vi "SwerveDriveFace.vi"(0 "Strafe Joystick Axes":cluster{"X":dbl, "Y":dbl}, 1 "Face Joystick Axes":cluster{"X":dbl, "Y":dbl}, 3 "Face PID Gains":T9 {"derivative time (Td, min)" format="%.3f"; "integral time (Ti, min)" format="%.3f"; "proportional gain (Kc)" format="%.3f"}, 4 "Angle (degrees; 0 = right)":dbl, 5 "error in (no error)":errorcluster, 6 "Strafe Multiplier":dbl, 7 "Steering Motor Refs":T1[](array[typedef]), 8 "Rotation Multiplier":dbl, 9 "Speed Motor Refs":T1[](array[typedef]), 10 "Max Wheel Speed":dbl) -> (14 "Steering Motor Setpoints":dbl[](array[numeric]), 15 "Speed Motor Setpoints":dbl[](array[numeric]), 16 "Speed Chart":cluster{dbl, "Encoder Velocity":dbl}[](graph), 19 "error out":errorcluster)   [LabVIEW 2015, in "Team900SwerveDrive.lvlib"]
uses:
  Team900SwerveDrive.lvlib
  <vilib>/Rock Robotics/WPI/MotorControl/WPI_MotorControlDeviceRef.ctl
  <vilib>/Rock Robotics/WPI/MotorControl/WPI_MotorControlType.ctl
  <vilib>/Rock Robotics/SystemInterfaces/DIO/FPGA_DIOPWMChannel.ctl
  <vilib>/Rock Robotics/WPI/PWM/WPI_PWMDeadband.ctl
  <vilib>/Rock Robotics/WPI/CAN/Jaguar/SubVIs/WPI_CANJaguar_ControlMode.ctl
  <vilib>/Rock Robotics/WPI/CAN/TalonSRX/WPI_CANTalonSRX_APIControlMode.ctl
  <vilib>/addons/control/pid/pid.llb/PID Control Input Filter (DBL).vi
  <vilib>/addons/control/pid/pid.llb/PID (DBL).vi
  <vilib>/addons/control/pid/NI_PID_pid.lvlib
panel:
  out "diff.":dbl
  out "Waveform Chart":T8(graph)
  out "Robot Heading":dbl(knob) scale=3.1416..-3.1416
  out "Joystick Angle":dbl(knob) scale=3.1416..-3.1416
  # "A version of SwerveDrive.vi which only takes\ntwo joysticks, one for strafe and one to use \nas a setpoint for angle"
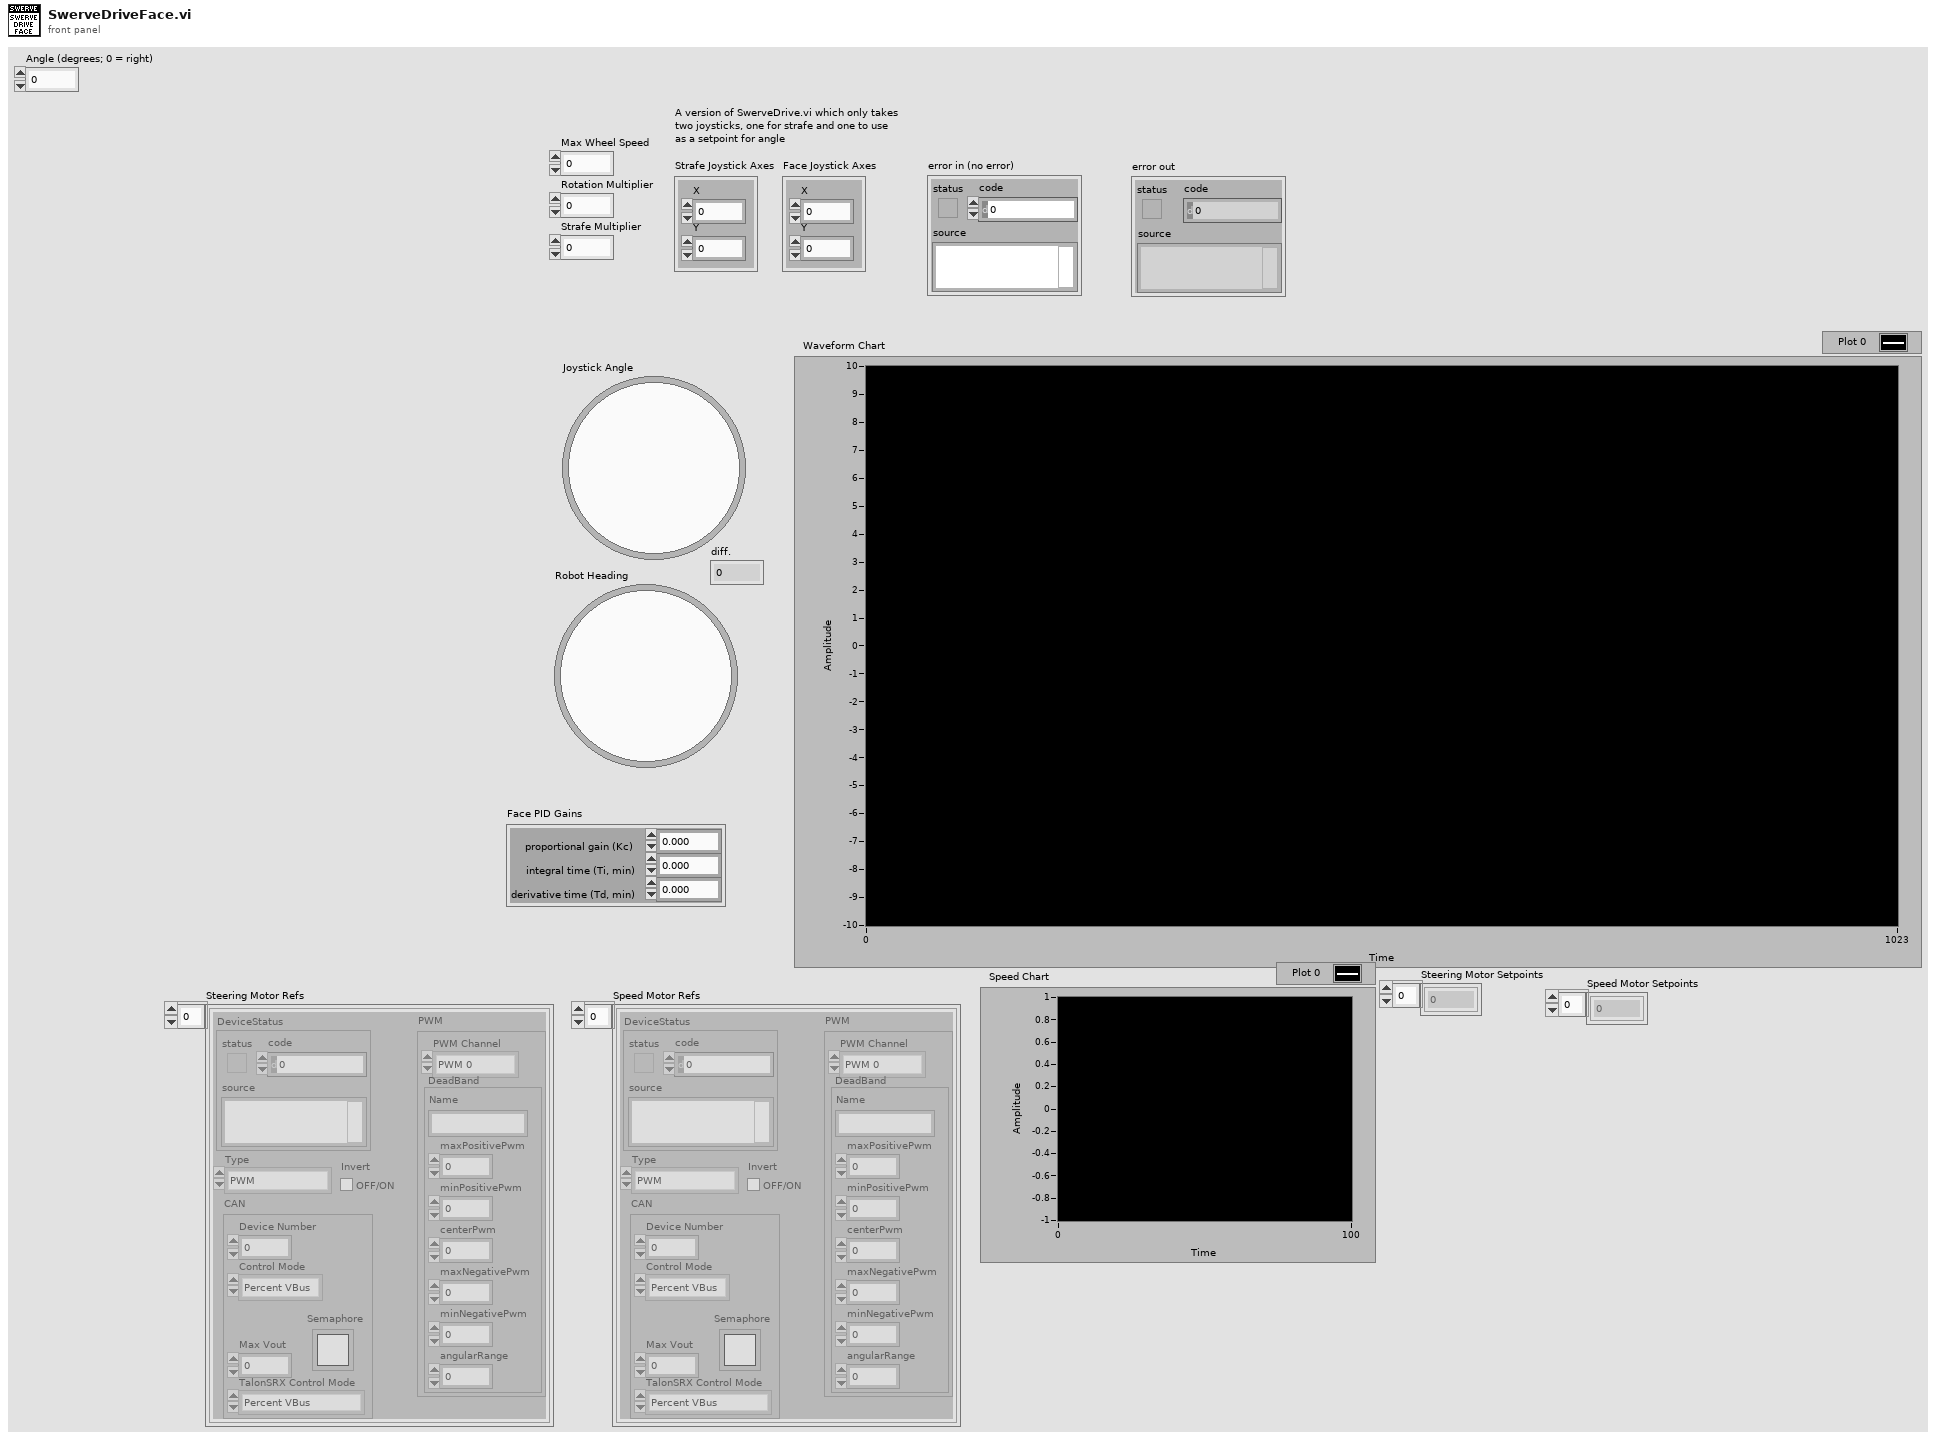
[diagram p1: front panel]
types:
  T1 = typedef "WPI_MotorControlDeviceRef.ctl" = cluster{"DeviceStatus":errorcluster, "Type":T2, "PWM":cluster{"PWM Channel":T3, "DeadBand":T4}, "CAN":cluster{"Device Number":u8, "Control Mode":T5, "Semaphore":T6, "Max Vout":dbl, "TalonSRX Control Mode":T7}, "Invert":bool}
  T2 = typedef "WPI_MotorControlType.ctl" = enum16{"PWM", "CAN", "CANTalonSRX"}
  T3 = typedef "FPGA_DIOPWMChannel.ctl" = enum8{"PWM 0", "PWM 1", "PWM 2", "PWM 3", "PWM 4", "PWM 5", "PWM 6", "PWM 7", "PWM 8", "PWM 9", "PWM MXP 0", "PWM MXP 1", "PWM MXP 2", "PWM MXP 3", "PWM MXP 4", "PWM MXP 5", "PWM MXP 6", "PWM MXP 7", "PWM MXP 8", "PWM MXP 9", "Invalid"}
  T4 = typedef "WPI_PWMDeadband.ctl" = cluster{"Name":string, "maxPositivePwm":i32, "minPositivePwm":i32, "centerPwm":i32, "maxNegativePwm":i32, "minNegativePwm":i32, "angularRange":u16}
  T5 = typedef "WPI_CANJaguar_ControlMode.ctl" = enum8{"Percent VBus", "Current", "Speed", "Position", "Voltage"}
  T6 = typedef "Semaphore RefNum" = refnum<k1>
  T7 = typedef "WPI_CANTalonSRX_APIControlMode.ctl" = enum8{"Percent VBus", "Speed", "Position", "Slave", "Unchanged / Invalid", "Voltage Compensation", "Current", "Motion Profile"}
  T8 = cluster{"output":dbl, "output":dbl, "millisecond timer value":u32}
  T9 = cluster{"proportional gain (Kc)":dbl, "integral time (Ti, min)":dbl, "derivative time (Td, min)":dbl}
  T10 = cluster{"output angle":dbl, "output":dbl, "millisecond timer value":u32}
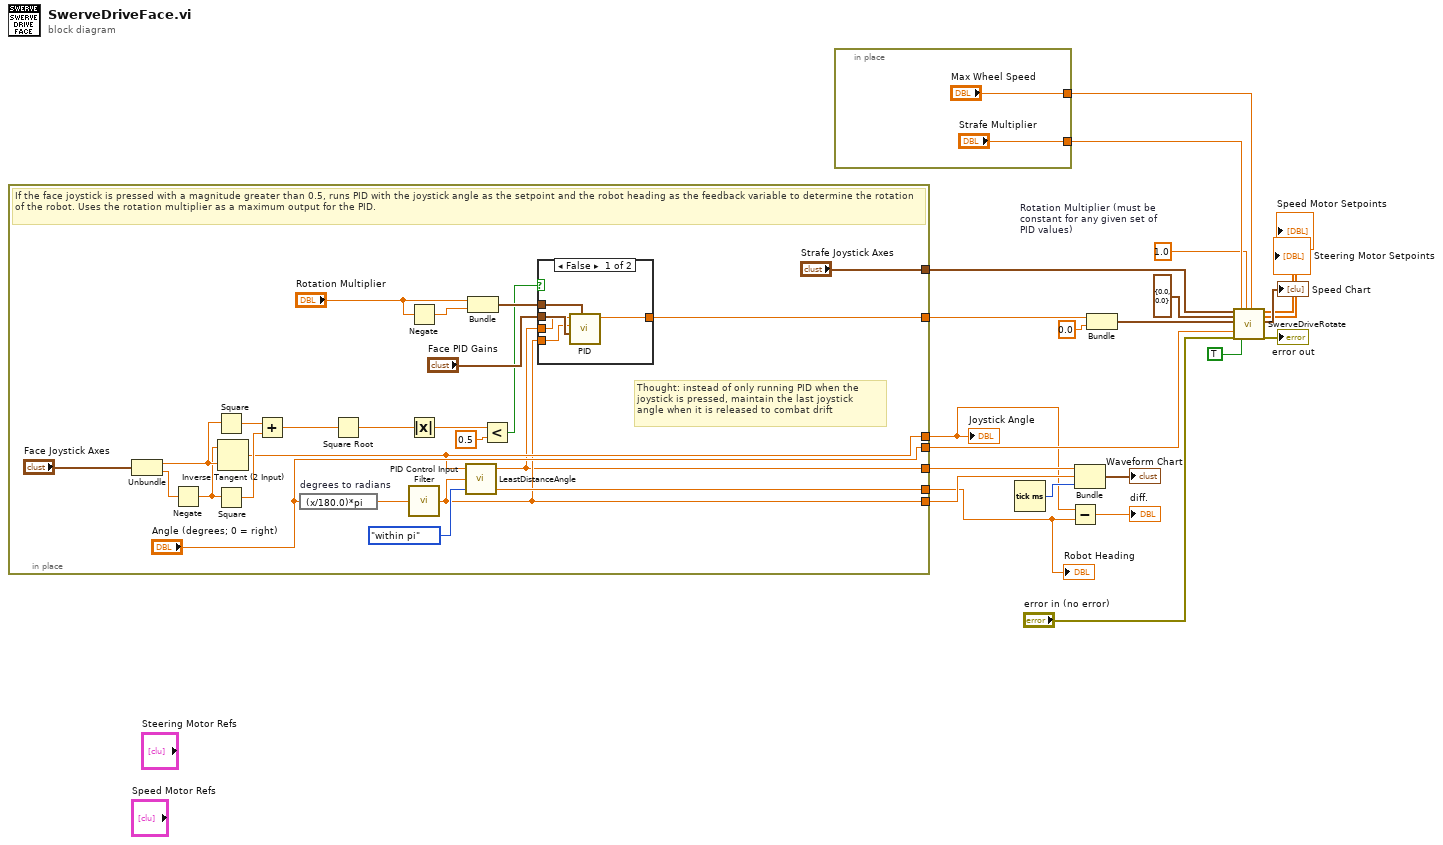
[diagram p0: block diagram]
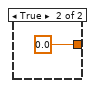
[diagram p2: hidden frame]
diagram:
  w10 = 1.0  # Rotation Multiplier (must be constant for any given set of PID values)
  n1 = in-place {
    in-place-border: [w46] -> w19
    in-place-border: ["Strafe Joystick Axes"] -> w22
    in-place-border: ["Angle (degrees; 0 = right)"] -> w18
    in-place-border: [w26] -> w7
    in-place-border: [w28] -> w6
    in-place-border: [w24] -> w9
    in-place-border: [w23] -> w8
    # "Thought: instead of only running PID when the\njoystick is pressed, maintain the last joystick\nangle when it is released to combat drift"
    # "If the face joystick is pressed with a magnitude greater than 0.5, runs PID with the joystick angle as the setpoint and the robot heading as the feedback variable to determine the rotation of the robot. Uses the rotation multiplier as a maximum output for the PID."
    n2 = Unbundle("Face Joystick Axes") -> ("X"=w38:dbl, "Y"=w37:dbl)
    n3 = Negate(x=w37) -> (-x=w32:dbl)
    n4 = Square(x=w38) -> (x^2=w42:dbl)
    n5 = Square(x=w32) -> (x^2=w41:dbl)
    n6 = Inverse Tangent (2 Input)(1:w38, 2:w32) -> (0:w26:dbl)
    n7 = Add(x=w42, y=w41) -> (x+y=w40:dbl)
    n8 = expression code="(x/180.0)*pi" "degrees to radians"("Angle (degrees; 0 = right)") -> (w43:dbl)
    n9 = Square Root(x=w40) -> (sqrt(x)=w39:dbl)
    n10 = Negate(x="Rotation Multiplier") -> (-x=w30:dbl)
    n11 = Absolute Value(x=w39) -> (abs(x)=w35:dbl)
    n12 = call-poly <vilib>:"PID Control Input Filter.vi"("input"=w43) -> ("output"=w24:dbl)  [unwired: 4 in]
    n13 = call "LeastDistanceAngle.vi"("Enum"=enum16{"within pi", "within pi/2"}."within pi", "Current angle"=w24, "target angle (between pi and -pi) 2"=w26) -> ("current angle (between pi and -pi) 2"=w28:dbl, "output angle"=w23:dbl)  [unwired: 1 out]
    n14 = Bundle("Rotation Multiplier"="Rotation Multiplier", w30) -> (w29:cluster{"Rotation Multiplier":dbl, dbl})  [unwired: 1 in]
    n15 = Less?(x=w35, y=0.5) -> (x < y?=w25:bool)
    n16 = case shown="False" w25 {
      tunnel: [w51 0.0 ("output")] -> w46
      tunnel: "Face PID Gains" -> [w50 _]
      tunnel: w29 -> [w49 _]
      tunnel: w24 -> [w48 _]
      tunnel: w23 -> [w47 _]
      frame False {
        n17 = call-poly <vilib>:"PID.vi"("output range"=w49, "PID gains"=w50, "process variable"=w48, "setpoint"=w47) -> ("output"=w51:dbl)  [unwired: 6 in, 1 out]
      }
      frame True {
      }
    }
  }
  "Joystick Angle" <- w7
  "Robot Heading" <- w6
  n18 = in-place {
    in-place-border: ["Max Wheel Speed"] -> w14
    in-place-border: ["Strafe Multiplier"] -> w11
  }
  n19 = Tick Count (ms)() -> (millisecond timer value=w13:u32)
  n20 = Subtract(x=w7, y=w6) -> (x-y=→"diff.":dbl)
  n21 = Bundle("output angle"=w8, "output"=w9, "millisecond timer value"=w13) -> (→"Waveform Chart":T10)  [unwired: 1 in]
  n22 = Bundle("output"=w19, 0.0) -> (w4:cluster{"output":dbl, dbl})  [unwired: 1 in]
  n23 = call "SwerveDriveRotate.vi"("Strafe Joystick Axes"=w22, "Center of Rotation Joystick Axes"=cluster{"X":dbl, "Y":dbl} {"X"=0.0, "Y"=0.0}, "Trigger Axes"=w4, "Angle (degrees; 0 = right)"=w18, "error in (no error)"="error in (no error)", "Strafe Multiplier"=w11, "FieldCentric? (T)"=TRUE, "Rotation Multiplier"=w10, "Max Wheel Speed"=w14) -> ("Steering Motor Setpoints"=→"Steering Motor Setpoints":dbl[], "Speed Motor Setpoints"=→"Speed Motor Setpoints":dbl[], "Speed Chart"=→"Speed Chart":cluster{dbl, "Encoder Velocity":dbl}[], "error out"=→"error out":errorcluster)  [unwired: 6 in, 1 out]
